vi "plot_XY.vi"(4 "exclude":dbl, 6 "exclude_where_x":bool caption="filter_inject", 7 "sort_by_x":bool caption="sort_x", 9 "Y_Data":dbl[](array[numeric]), 10 "X_Data":dbl[](array[numeric])) -> (2 "XY Graph":cluster{"sorted_x":dbl[], "sorted_y ":dbl[]}[](graph))   [LabVIEW 2017, in "tools.lvlib"]
uses:
  tools.lvlib
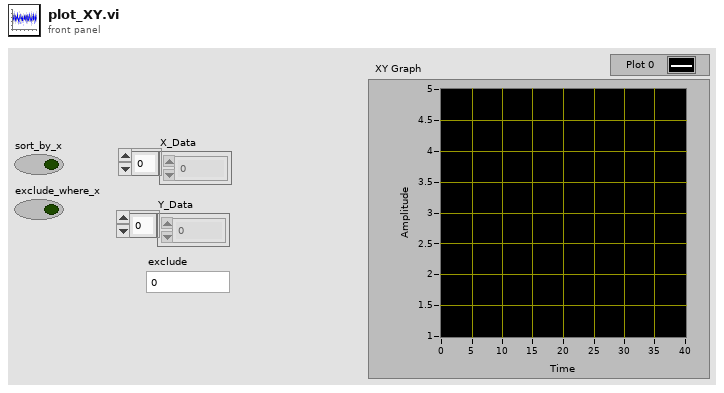
[diagram p1: front panel]
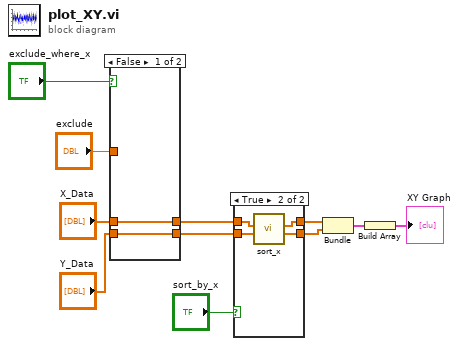
[diagram p0: block diagram]
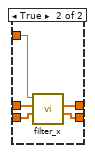
[diagram p3: hidden frame]
diagram:
  n1 = case shown="False" "exclude_where_x" {
    tunnel: [w13 w18] -> w11
    tunnel: [w12 w17] -> w10
    tunnel: "exclude" -> [_ w16]
    tunnel: "X_Data" -> [w13 w15]
    tunnel: "Y_Data" -> [w12 w14]
    frame False {
    }
    frame True {
      n2 = call "filter_x.vi"("y"=w14, "x"=w15, "exclude_where_x"=w16) -> ("filtered_y"=w17:dbl[], "filtered_x"=w18:dbl[])  [unwired: 7 in]
    }
  }
  n3 = case shown="True" "sort_by_x" {
    tunnel: [w20 w22] -> w8
    tunnel: w11 -> [w20 w24]
    tunnel: w10 -> [w19 w23]
    tunnel: [w19 w21] -> w9
    frame False {
    }
    frame True {
      n4 = call "sort_x.vi"("y"=w23, "x"=w24) -> ("sorted_y"=w21:dbl[], "sorted_x"=w22:dbl[])  [unwired: 8 in]
    }
  }
  n5 = Bundle("sorted_x"=w8, "sorted_y"=w9) -> (w2:cluster{"sorted_x":dbl[], "sorted_y ":dbl[]})  [unwired: 1 in]
  n6 = Build Array(w2) -> (→"XY Graph":cluster{"sorted_x":dbl[], "sorted_y ":dbl[]}[])
